vi "niFPGA SQRT Integer (48 bit) - Rounded.vi"(4 "x [U64]":u64 format="%.0x") -> (1 "sqrt (x) [U32]":u32 format="%.0x")   [LabVIEW 2017]
doc: "Iteratively computes the rounded integer square root of an unsigned 48-bit input using a binary restoring square root extraction algorithm. The rounding mode is round to nearest (+Inf), in which one extra bit is computed to determine whether to round up or down.\n\nNOTE: Input values must be less than (2^24 - .5)^2 (ie, less than or equal to xFFFFFF000000) in order to avoid overflowing the computed 24-bit output integer. Overflow will result in an output of 2^24, or x1000000."
uses:
  <vilib>/Platform/TimedLoop/XDataNode/timing_clust.ctl
  <vilib>/Platform/TimedLoop/XDataNode/nitl_modes.ctl
  <vilib>/Platform/TimedLoop/XDataNode/wakeup.ctl
  <vilib>/Platform/TimedLoop/XDataNode/XDataNode.xnode
  <vilib>/Platform/TimedLoop/XDataNode/XDNodeRunTimeDep.lvlib
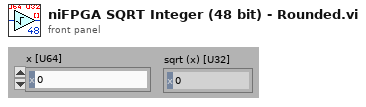
[diagram p1: front panel]
types:
  T1 = typedef "XDNodeRunTimeDep.lvlib/timing_clust.ctl" = cluster{"Expected End [f-1]":u64, "Actual End [f-1]":u64, "Finished Late? [f-1]":bool, "Expected End [i-1]":u64, "Actual End [i-1]":u64, "Finished Late? [i-1]":bool, "Expected Start [i]":u64, "Actual Start [i]":u64, "Expected Start [f]":u64, "Actual Start [f]":u64, "Source Name":string, "Structure Name":string, "Period":i64, "Deadline":i64, "Offset":i64, "Start":i64, "Priority":i32, "Timeout":i32, "Mode":T2, "Wakeup Reason":T3, "Error":errorcluster, "Source Type":string, "Secondary Source Type":string, "Global End Time":u64, "Global Start Time":u64, "Frame Duration":u64, "Iteration Duration":u64, "Assigned CPU":i32, "I/O Scan Engine Mode":u32}
  T2 = typedef "XDNodeRunTimeDep.lvlib/nitl_modes.ctl" = enum32{"No Change", "Process missed periods, maintain original phase", "Discard missed periods, maintain original phase", "Process missed periods, ignore original phase", "Discard missed periods, ignore original phase"}
  T3 = typedef "XDNodeRunTimeDep.lvlib/wakeup.ctl" = enum32{"Normal", "Aborted", "Asynchronous wakeup", "Timing source error", "Timed loop error", "Timeout"}
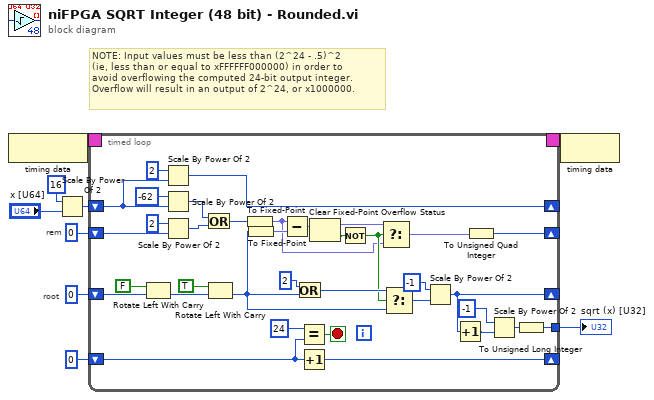
[diagram p0: block diagram]
diagram:
  # "NOTE: Input values must be less than (2^24 - .5)^2 \n(ie, less than or equal to xFFFFFF000000) in order to \navoid overflowing the computed 24-bit output integer. \nOverflow will result in an output of 2^24, or x1000000."
  # "rem"
  # "root"
  n1 = node-c288() -> (w2:T1)
  n2 = Scale By Power Of 2(n=i8 16, x="x [U64]") -> (x*2^n=w6:u64)
  n3 = timed-loop {
    shift-left: u64 0 ("x [U32.2]") -> [w36]
    shift-right: [w14] -> _
    shift-left: u64 0 ("x [U32.2]") -> [w44]
    shift-right: [w16] -> _
    shift-left: w6 -> [w41]
    shift-right: [w37] -> _
    tunnel: [w15] -> w3
    shift-right: [w20] -> _
    shift-left: u8 0 -> [w21]
    timing: w2 -> [_]
    timing-out: [_] -> w1
    stop <- w19 stop-if-true
    n4 = Rotate Left With Carry(2:w44, 3:FALSE ("carry")) -> (0:w33:u64)  [unwired: 1 out]
    n5 = Scale By Power Of 2(n=i8 2, x=w41) -> (x*2^n=w37:u64)
    n6 = Scale By Power Of 2(n=i8 -62, x=w41) -> (x*2^n=w39:u64)
    n7 = Scale By Power Of 2(n=i8 2, x=w36) -> (x*2^n=w35:u64)
    n8 = Or(x=w39, y=w35) -> (x .or. y?=w25:u64)
    n9 = Rotate Left With Carry(2:w33, 3:TRUE ("carry")) -> (0:w28:u64)  [unwired: 1 out]
    n10 = To Fixed-Point(number=w25) -> (fixed-point=w10:fxp<+,64,64>)  [unwired: 1 out]
    n11 = To Fixed-Point(number=w28) -> (fixed-point=w13:fxp<+,64,64>)  [unwired: 1 out]
    n12 = Subtract(x=w10, y=w13) -> (x-y=w26:fxp<+,64,64>)
    n13 = Or(x=u64 2, y=w28) -> (x .or. y?=w30:u64)
    n14 = Equal?(x=u8 24, y=w21) -> (x = y?=w19:bool)
    n15 = Increment(x=w21) -> (x+1=w20:u8)
    n16 = Clear Fixed-Point Overflow Status(3:w26) -> (0:w11:bool, 1:w12:fxp<+,64,64>)
    n17 = Not(x=w11) -> (.not. x?=w27:bool)
    n18 = Select(t=w12, s=w27, f=w10) -> (s? t:f=w24:fxp<+,64,64>)
    n19 = Select(t=w30, s=w27, f=w28) -> (s? t:f=w29:u64)
    n20 = Scale By Power Of 2(n=i8 -1, x=w29) -> (x*2^n=w16:u64)
    n21 = Increment(x=w16) -> (x+1=w17:u64)
    n22 = To Unsigned Quad Integer(1:w24) -> (0:w14:u64)
    n23 = Scale By Power Of 2(n=i8 -1, x=w17) -> (x*2^n=w18:u64)
    n24 = To Unsigned Long Integer(number=w18) -> (unsigned 32bit integer=w15:u32)
  }
  "sqrt (x) [U32]" <- w3
  n25 = node-c288(w1) -> ()
